vi "default file paths.vi"() -> (2 "paths":T1)   [LabVIEW 2013, in "configuration library.lvlib"]
uses:
  configuration library.lvlib
  Controls/FilePaths.ctl
  <vilib>/Utility/libraryn.llb/Check if File or Folder Exists.vi
  <vilib>/NI/Tag Bus Data Framework/Framework Configuration Classes/class cache/PL_class cache.lvlib
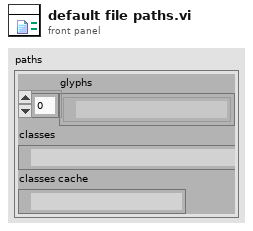
[diagram p1: front panel]
types:
  T1 = typedef "configuration library.lvlib/FilePaths.ctl" = cluster{"glyphs":path[], "classes":path, "classes cache":path}
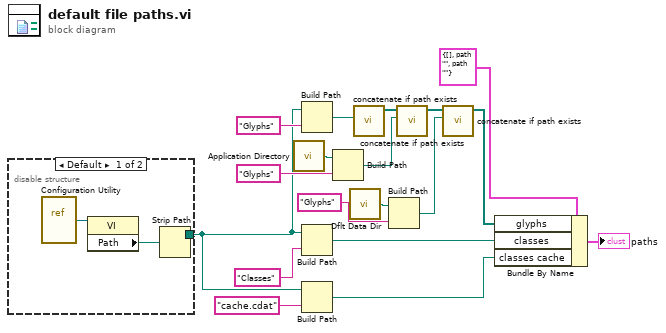
[diagram p0: block diagram]
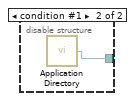
[diagram p2: hidden frame]
diagram:
  n1 = disable-structure shown="Default" {
    disable-tunnel: [w21 w22] -> w1
    frame condition #0 (active) {
      n2 = vi-ref "Configuration Utility.vi"() -> (w20:refnum<vi>)
      n3 = property class="VI"(reference=w20) -> ("Path"=w19:path)  [unwired: 1 in, 2 out]
      n4 = Strip Path(path=w19) -> (stripped path=w21:path)  [unwired: 1 out]
    }
    frame condition #1 {
      n5 = call <vilib>:"Application Directory.vi"() -> ("Application Directory"=w22:path)
    }
  }
  n6 = call <vilib>:"Application Directory.vi"() -> ("Application Directory"=w13:path)
  n7 = Build Path(base path=w1, name or relative path="Glyphs") -> (appended path=w2:path)
  n8 = Build Path(base path=w1, name or relative path="Classes") -> (appended path=w14:path)
  n9 = Build Path(base path=w1, name or relative path="cache.cdat") -> (appended path=w11:path)
  n10 = Build Path(base path=w13, name or relative path="Glyphs") -> (appended path=w7:path)
  n11 = call <vilib>:"Dflt Data Dir.vi"() -> ("App:Default Data Directory"=w9:path)
  n12 = call <vilib>:"concatenate if path exists.vi"("new path"=w2) -> ("paths out"=w3:path[])  [unwired: 10 in]
  n13 = Build Path(base path=w9, name or relative path="Glyphs") -> (appended path=w8:path)
  n14 = call <vilib>:"concatenate if path exists.vi"("new path"=w7, "paths in"=w3) -> ("paths out"=w6:path[])  [unwired: 9 in]
  n15 = call <vilib>:"concatenate if path exists.vi"("new path"=w8, "paths in"=w6) -> ("paths out"=w5:path[])  [unwired: 9 in]
  n16 = Bundle By Name(cluster=T1 {"glyphs"=[], "classes"=path "", "classes cache"=path ""} ("Cluster 2"), "glyphs"=w5, "classes"=w14, "classes cache"=w11) -> (→"paths":T1)
